vi "new itc and dmm file 2.vi"() -> ()   [LabVIEW 2009]
panel:
  out "Waveform Chart":dbl(graph)
  out "source out 2":string
  out "message 2":string
  out "error out 2":errorcluster
  out "error? 2":bool
  out "Sensor Resistance 2":dynamicdata(graph)
  out "Sensors Temperature 2":dynamicdata(graph)
  out "Resistance 2":dynamicdata(graph)
  out "Temperature 2":dynamicdata(graph)
  in  "stop 2":bool
  out "Measurement":bool caption="Taken"
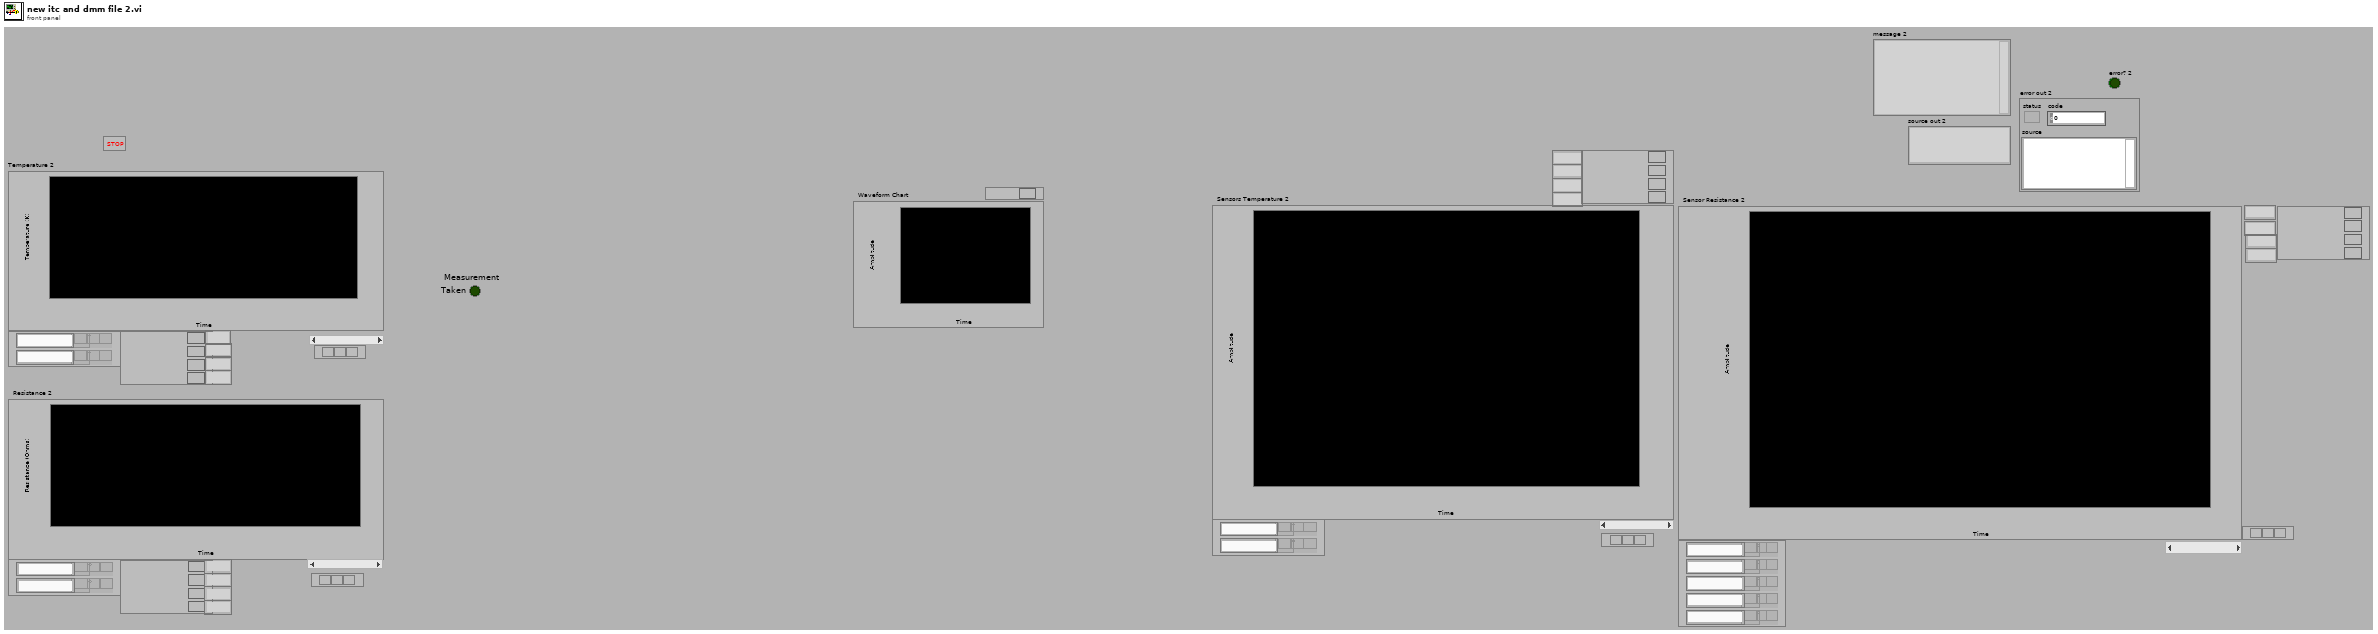
[diagram p1: front panel]
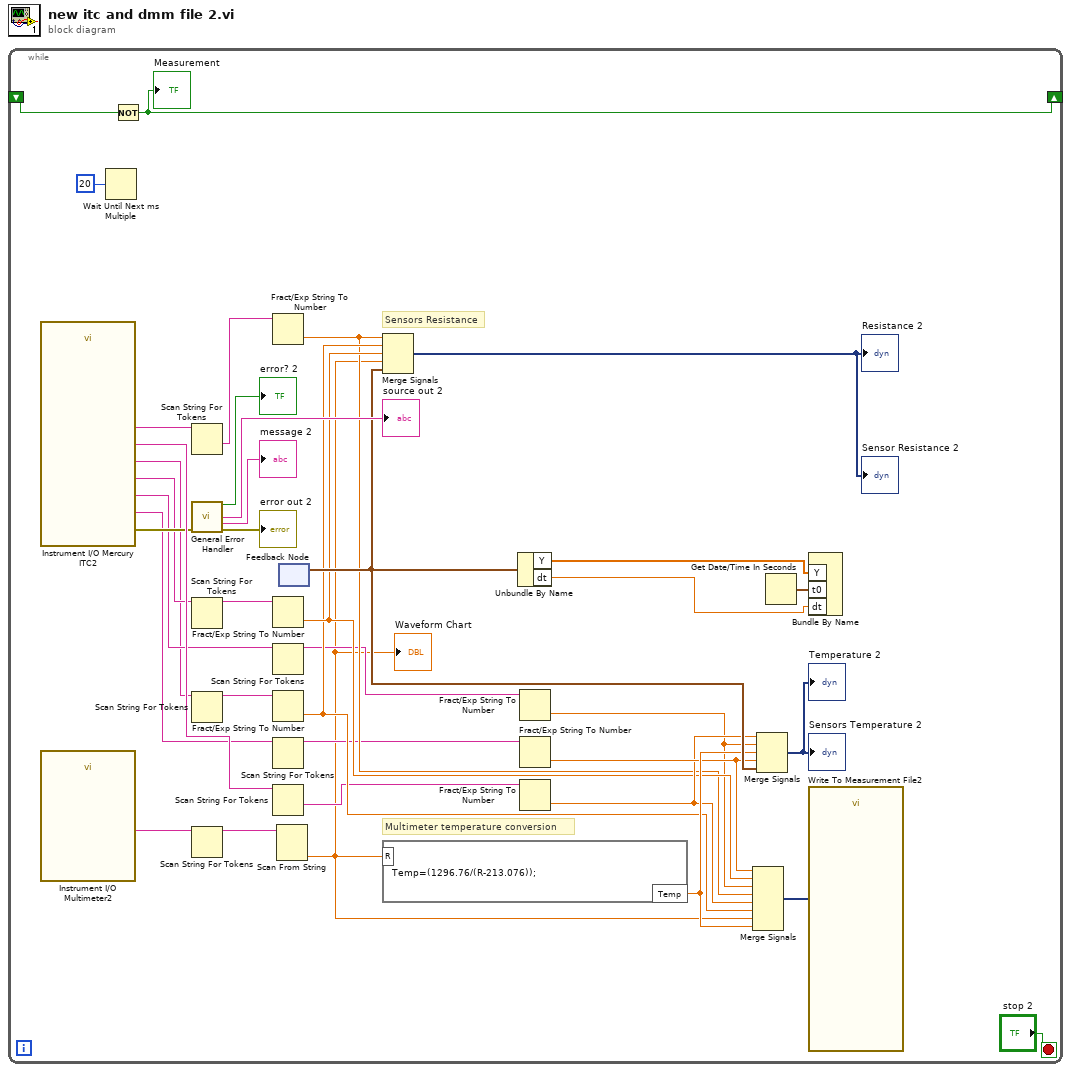
[diagram p0: block diagram]
diagram:
  n1 = while {
    shift-right: [w38] -> _
    shift-left: _ -> [w39]
    stop <- "stop 2" stop-if-true
    # "Sensors Resistance"
    # "Multimeter temperature conversion"
    n2 = call "Instrument I/O Mercury ITC2"() -> ("CCS Resistance"=w13:string, "CCS Temperature"=w15:string, "Allen Bradley Temperature"=w11:string, "Allen Bradley Resistance"=w9:string, "Cernox Temp"=w36:string, "Cernox Resistance"=w4:string, "error out"=w30:errorcluster)  [unwired: 21 in]
    n3 = call "Instrument I/O Multimeter2"() -> ("Sample rate"=w35:string)  [unwired: 25 in, 2 out]
    n4 = Wait Until Next ms Multiple(millisecond multiple=u32 20) -> ()  [unwired: 1 out]
    n5 = Not(x=w39) -> (.not. x?=w38:bool)
    "Measurement" <- w38
    n6 = Scan String For Tokens(9:w4) -> (1:w5:string)  [unwired: 5 in, 3 out]
    n7 = call <vilib>:"General Error Handler.vi"("error in (no error)"=w30) -> ("error?"=→"error? 2":bool, "source out"=→"source out 2":string, "message"=→"message 2":string, "error out"=→"error out 2":errorcluster)  [unwired: 10 in, 1 out]
    n8 = Scan String For Tokens(9:w13) -> (3:w14:string)  [unwired: 5 in, 3 out]
    n9 = Scan String For Tokens(9:w9) -> (3:w10:string)  [unwired: 5 in, 3 out]
    n10 = Scan String For Tokens(9:w35) -> (3:w17:string)  [unwired: 5 in, 3 out]
    n11 = Fract/Exp String To Number(string=w5) -> (number=w18:dbl)  [unwired: 3 in, 1 out]
    n12 = Fract/Exp String To Number(string=w14) -> (number=w20:dbl)  [unwired: 3 in, 1 out]
    n13 = Scan String For Tokens(9:w11) -> (3:w12:string)  [unwired: 5 in, 3 out]
    n14 = Fract/Exp String To Number(string=w10) -> (number=w19:dbl)  [unwired: 3 in, 1 out]
    n15 = Scan String For Tokens(9:w15) -> (3:w16:string)  [unwired: 5 in, 3 out]
    n16 = Scan String For Tokens(9:w36) -> (1:w7:string)  [unwired: 5 in, 3 out]
    n17 = Scan From String(input string=w17) -> (output 1=w2:dbl)  [unwired: 4 in, 3 out]
    "Waveform Chart" <- w2
    n18 = feedback #1() -> (w27:waveform(dbl))  [unwired: 1 in]
    n19 = Merge Signals(w18, w19, w20, w2, w27) -> (→"Resistance 2" →"Sensor Resistance 2":dynamicdata)
    n20 = formula code="Temp=(1296.76/(R-213.076));"("R"=w2) -> ("Temp"=w23:dbl)
    n21 = Unbundle By Name(w27) -> ("Y"=w24:dbl[], "dt"=w25:dbl)
    n22 = Fract/Exp String To Number(string=w12) -> (number=w3:dbl)  [unwired: 3 in, 1 out]
    n23 = Fract/Exp String To Number(string=w16) -> (number=w22:dbl)  [unwired: 3 in, 1 out]
    n24 = Fract/Exp String To Number(string=w7) -> (number=w21:dbl)  [unwired: 3 in, 1 out]
    n25 = Merge Signals(w22, w20, w3, w18, w21, w19, w2, w23) -> (w6:dynamicdata)
    n26 = Merge Signals(w21, w3, w23, w22, w27) -> (→"Temperature 2" →"Sensors Temperature 2":dynamicdata)
    n27 = Get Date/Time In Seconds() -> (seconds since 1Jan1904=w8:timestamp)
    n28 = Bundle By Name("Y"=w24, "t0"=w8, "dt"=w25) -> (w26:waveform(dbl))  [unwired: 1 in]
    n29 = call "Write To Measurement File2"("Signals"=w6) -> ()  [unwired: 16 in, 3 out]
  }
